vi "main 5th.vi"() -> ()   [LabVIEW 2015]
panel:
  out "data":u16[](array[numeric])
  out "size(s)":i32
  in  "bstrFilename":string
  out "Array":u16[][](array[numeric])
  out "element":u16[][](array[numeric])
  out "From OD fit?":bool
  in  "Current file num":i32
  in  "Fitting Results Save Path":string[](array[string])
  in  "Initial guess values":dbl[](array[numeric])
  out "Latest image data":dbl[][](array[numeric])
  in  "Fitting Type":u16(ring)
  in  "Force Guess?":bool
  out "x-y":u32
  out "best fit parameters":dbl[](array[numeric])
  in  "Reset process index":bool
  out "ROI Height":u32
  out "ROI Width":u32
  out "OD image":u16[][](graph)
  out "Process Index":i32
  out "External Trigger":bool
  out "XY图":cluster{i32[], dbl[]}[](graph)
  in  "OD fit":bool
  in  "OD num":i32
  out "Fit Done":bool
  in  "Exit":bool
  out "XY图 2":cluster{i32[], dbl[]}[](graph)
  in  "Fit":bool
  in  "Open File":bool
  in  "Auto Fit":bool
  in  "Stop":bool
  in  "Aquire":bool
  in  "Fitting Config":bool
  in  "Camera Config":bool
  in  "Initialize":bool
  in  "Live Image Display":refnum<k7>(container)
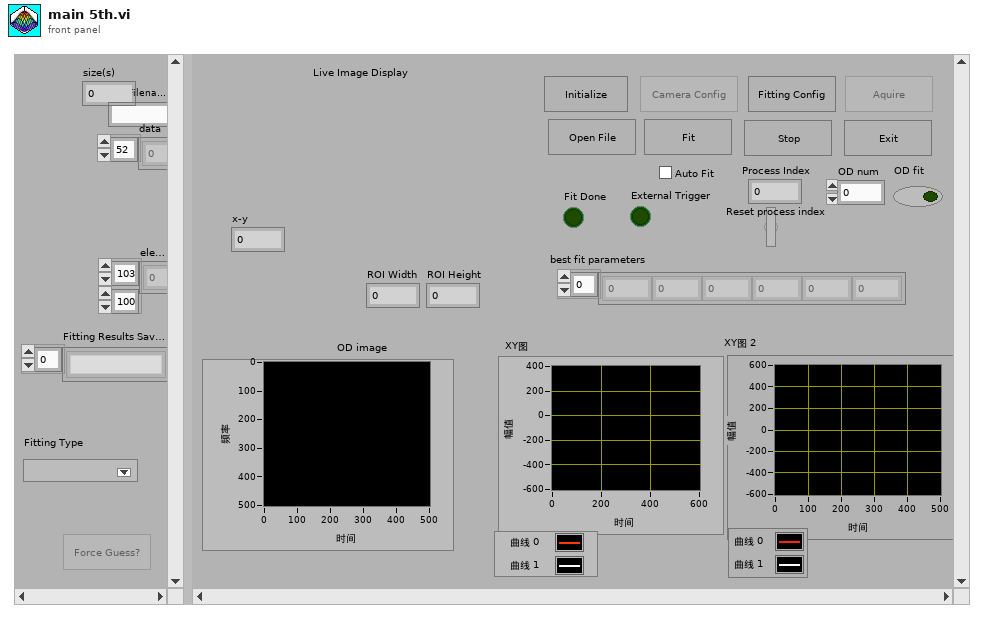
[diagram p1: front panel]
types:
  T1 = enum8{"Enabled", "Disabled", "Disabled and Grayed Out"}
  T2 = typedef "Image Type" = u32
  T3 = typedef "IMAQ Image.ctl" = refnum<image>
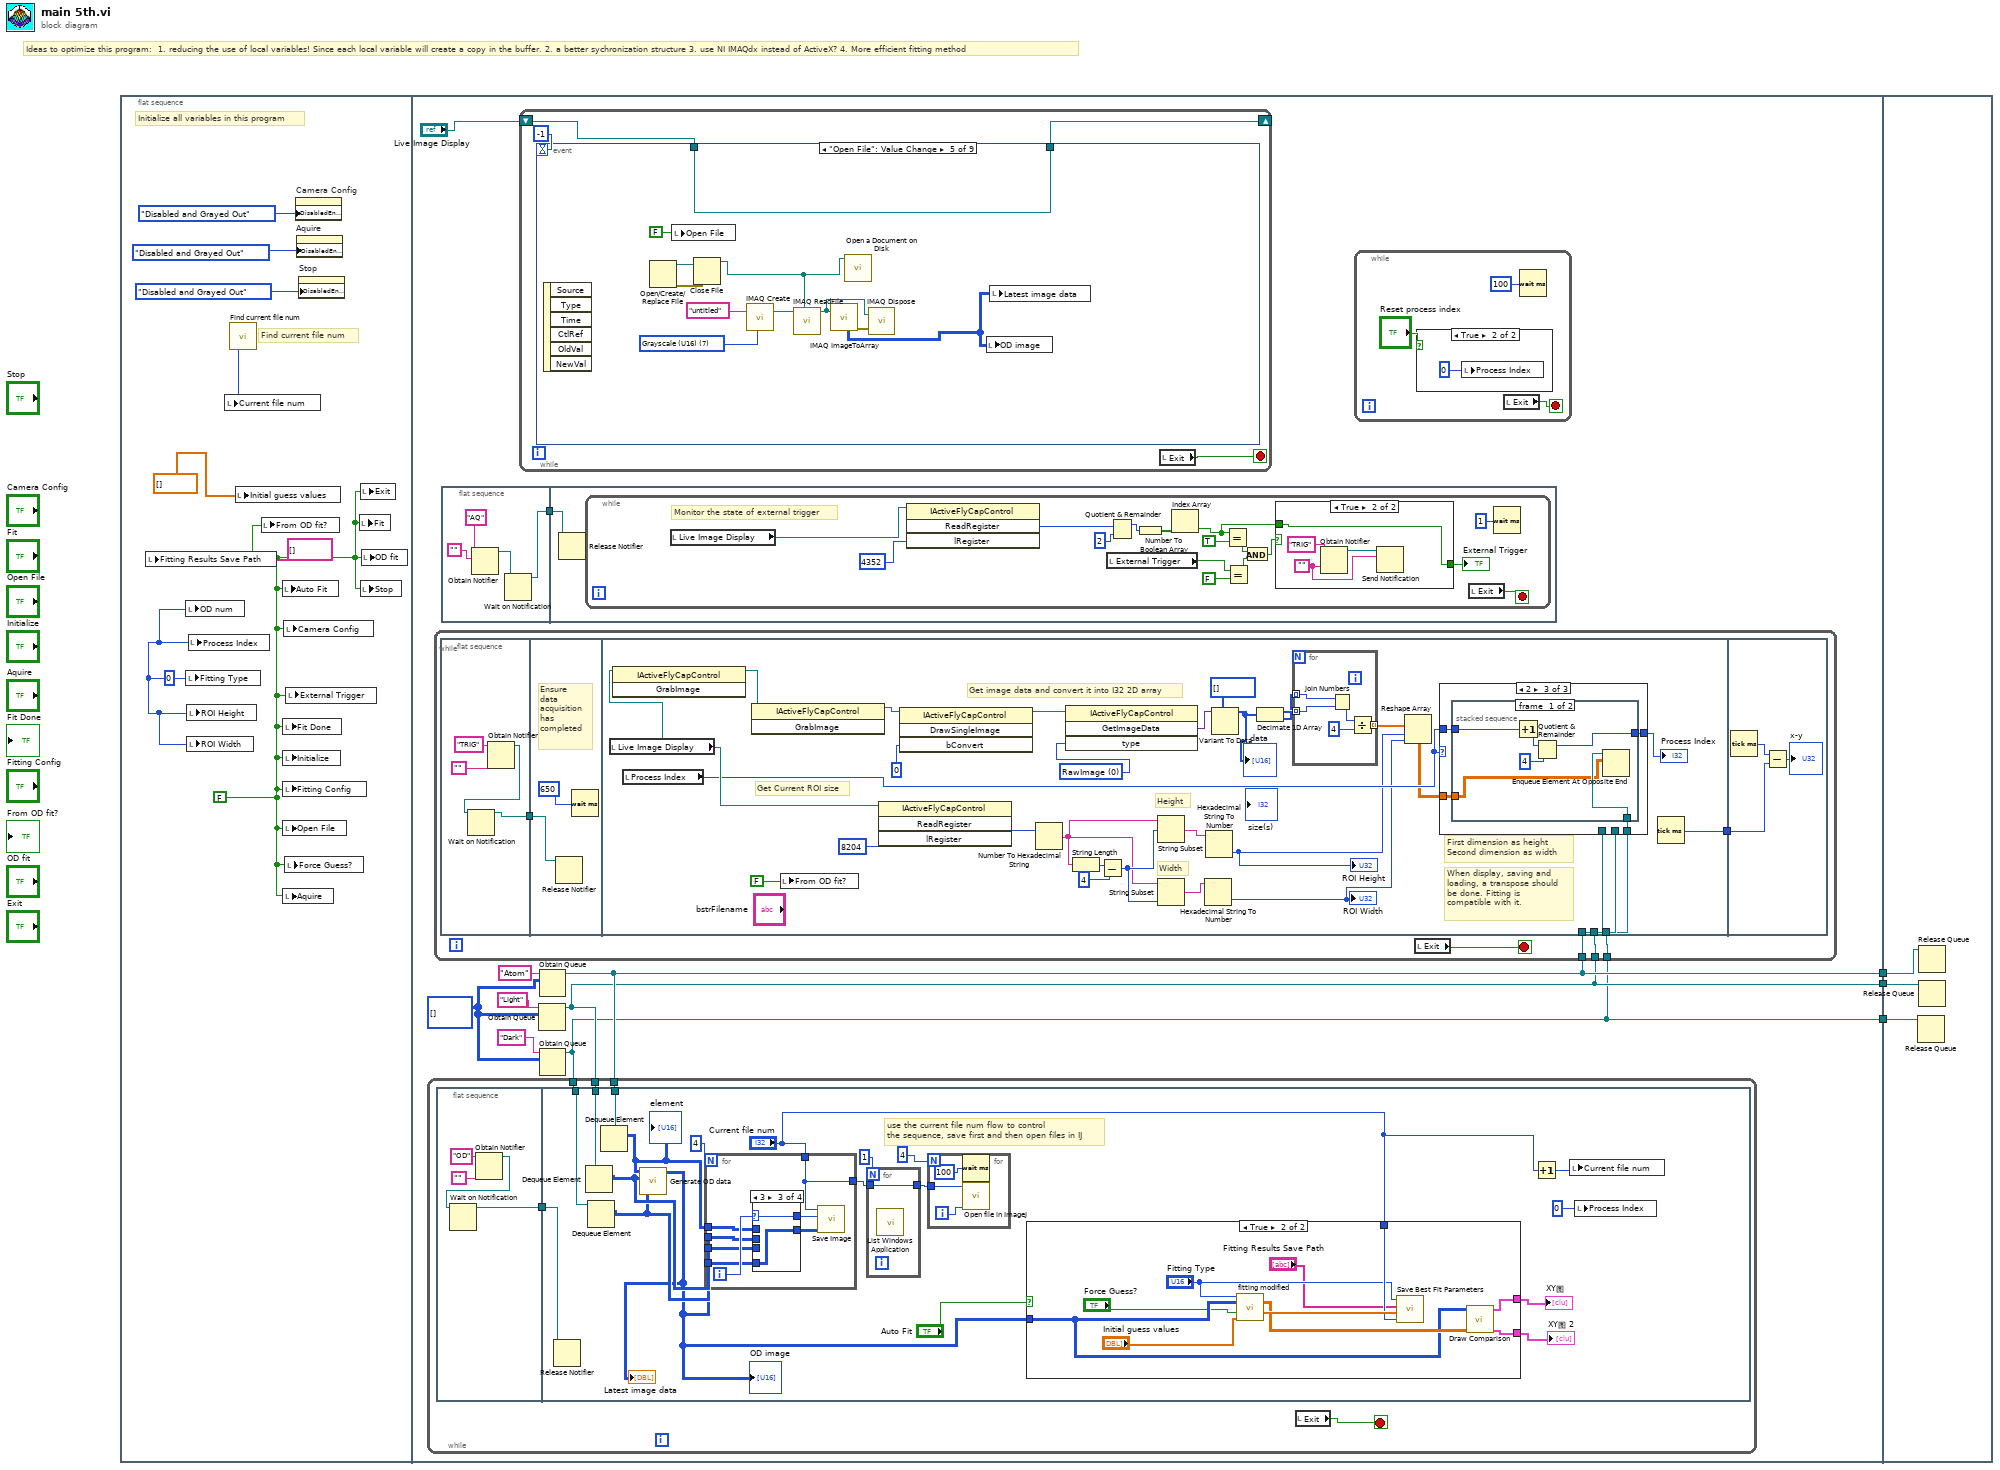
[diagram p0: block diagram]
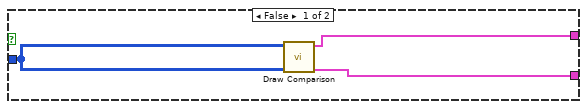
[diagram p3: hidden frame]
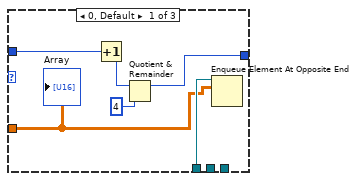
[diagram p8: hidden frame]
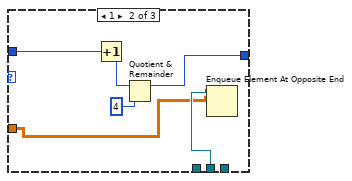
[diagram p9: hidden frame]
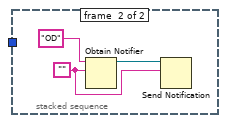
[diagram p10: hidden frame]
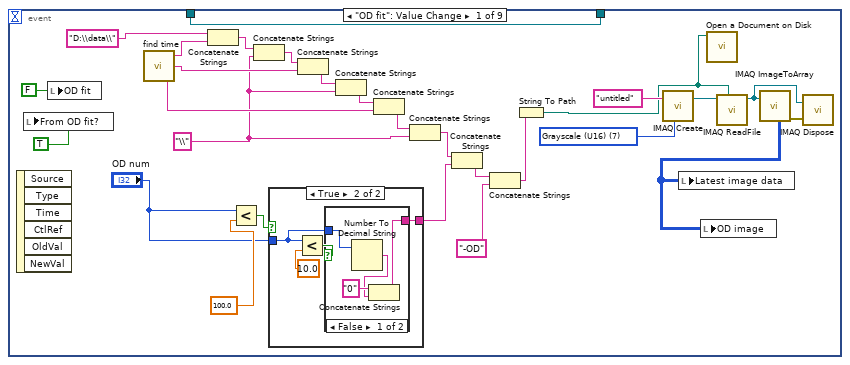
[diagram p11: hidden frame]
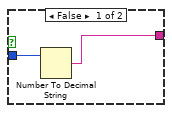
[diagram p12: hidden frame]
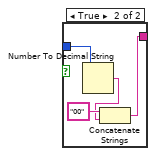
[diagram p13: hidden frame]
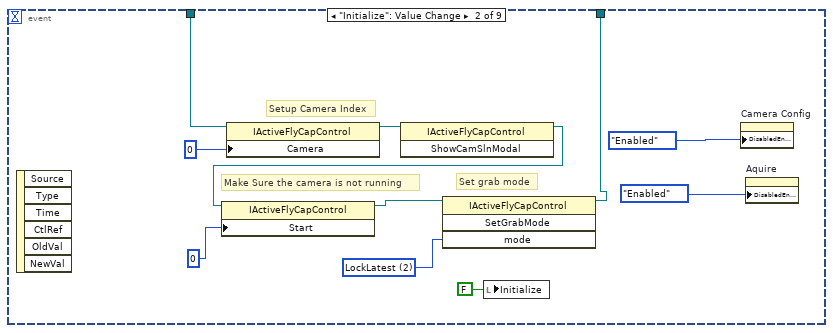
[diagram p14: hidden frame]
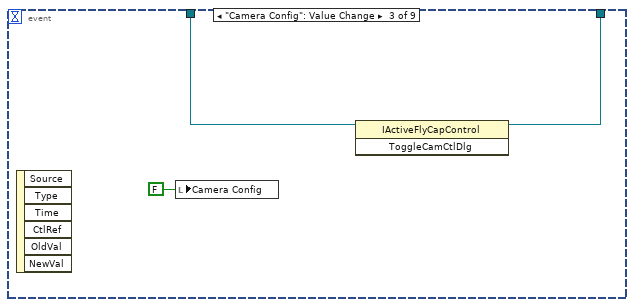
[diagram p15: hidden frame]
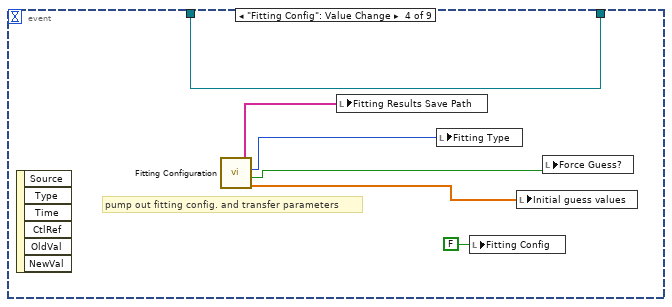
[diagram p16: hidden frame]
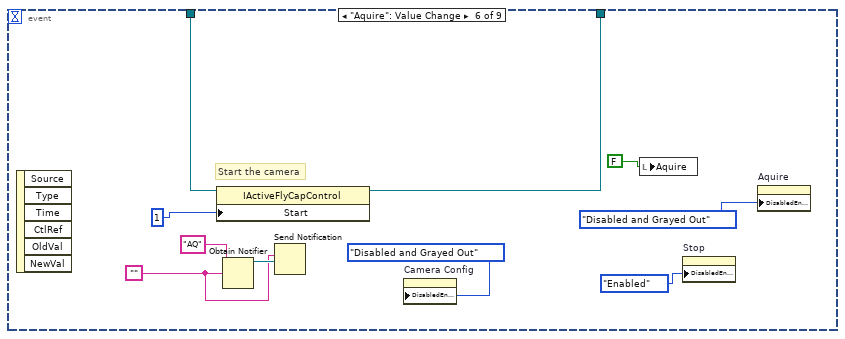
[diagram p17: hidden frame]
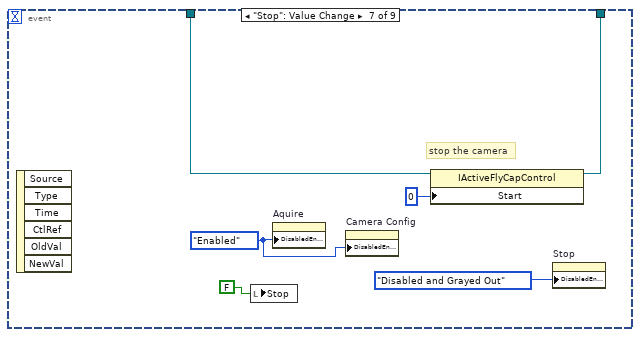
[diagram p18: hidden frame]
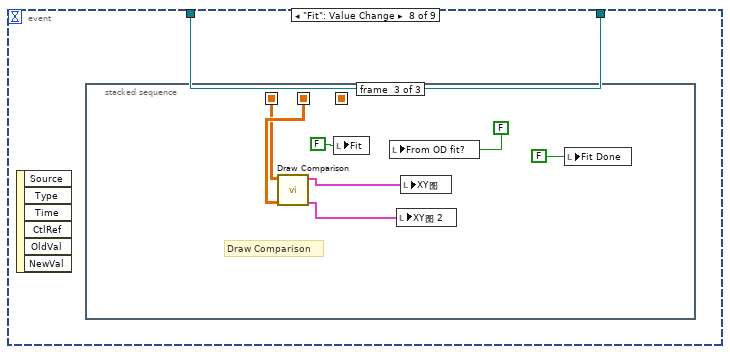
[diagram p19: hidden frame]
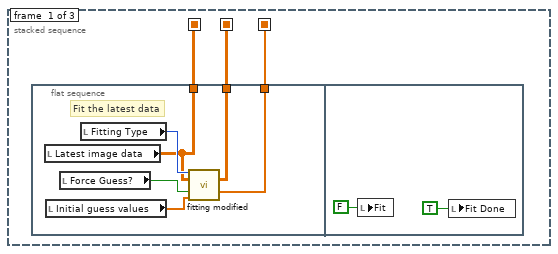
[diagram p20: hidden frame]
diagram:
  # "Ideas to optimize this program:  1. reducing the use of local variables! Since each local variable will create a copy in the buffer. 2. a better sychronization structure 3. use NI IMAQdx instead of ActiveX? 4. More efficient fitting method"
  n1 = flat-sequence {
    tunnel: [w15] -> w3
    tunnel: [w14] -> w2
    tunnel: [w13] -> w1
    tunnel: w3 -> [w309]
    tunnel: w2 -> [w308]
    tunnel: w1 -> [w307]
    frame #0 {
      w7 = 0 ("OD num")
      w5 = FALSE ("Aquire")
      # "Find current file num"
      # "Initialize all variables in this program"
      n2 = local write "Fitting Results Save Path"(string[] [] ("Fitting Results Save Path")) -> ()
      n3 = local write "OD num"(w7) -> ()
      n4 = local write "Fitting Type"(w7) -> ()
      n5 = local write "ROI Height"(w7) -> ()
      n6 = local write "ROI Width"(w7) -> ()
      n7 = local write "Process Index"(w7) -> ()
      n8 = call "Find current file num.vi"() -> ("Current File Num"=w4:u16)  [unwired: 2 in]
      n9 = local write "Current file num"(w4) -> ()
      n10 = local write "Initial guess values"(dbl[] [] ("Best fit parameters")) -> ()
      n11 = local write "From OD fit?"(w5) -> ()
      n12 = local write "Auto Fit"(w5) -> ()
      n13 = local write "Fit Done"(w5) -> ()
      n14 = local write "Initialize"(w5) -> ()
      n15 = local write "Fitting Config"(w5) -> ()
      n16 = local write "Open File"(w5) -> ()
      n17 = local write "Aquire"(w5) -> ()
      n18 = local write "Camera Config"(w5) -> ()
      n19 = local write "Force Guess?"(w5) -> ()
      n20 = local write "External Trigger"(w5) -> ()
      n21 = property on="Camera Config" class="Bool (strict)"("DisabledEnum"=T1."Disabled and Grayed Out" ("禁用")) -> ()  [unwired: 2 in, 2 out]
      n22 = property on="Aquire" class="Bool (strict)"("DisabledEnum"=T1."Disabled and Grayed Out" ("禁用")) -> ()  [unwired: 2 in, 2 out]
      n23 = property on="Stop" class="Bool (strict)"("DisabledEnum"=T1."Disabled and Grayed Out" ("禁用")) -> ()  [unwired: 2 in, 2 out]
      n24 = local write "Fit"(w5) -> ()
      n25 = local write "Exit"(w5) -> ()
      n26 = local write "Stop"(w5) -> ()
      n27 = local write "OD fit"(w5) -> ()
    }
    frame #1 {
      w16 = i32[][] [] ("输出数组")
      n28 = flat-sequence {
        tunnel: [w86] -> w20
        tunnel: w20 -> [w90]
        frame #0 {
          n29 = Obtain Notifier(name (unnamed)="AQ" ("名称（未命名）"), notification data type="") -> (notifier out=w88:refnum<notifier>)  [unwired: 2 in, 2 out]
          n30 = Wait on Notification(notifier=w88) -> (notifier out=w86:refnum<notifier>)  [unwired: 3 in, 3 out]
        }
        frame #1 {
          n31 = Release Notifier(notifier=w90) -> ()  [unwired: 2 in, 3 out]
          n32 = while {
            stop <- w106 stop-if-true
            # "Monitor the state of external trigger"
            n33 = local read "Live Image Display"() -> (w105:refnum<k7>)
            n34 = invoke class="IActiveFlyCapControl" method="ReadRegister"(reference=w105, "lRegister"=u32 4352) -> ("ReadRegister"=w103:u32)  [unwired: 2 in, 3 out]
            n35 = local read "External Trigger"() -> (w98:bool)
            n36 = Quotient & Remainder(x=w103, y=u32 2) -> (x-y*floor(x/y)=w101:u32)  [unwired: 1 out]
            n37 = Number To Boolean Array(number=w101) -> (Boolean array=w100:bool[])
            n38 = Index Array(array=w100) -> (element=w93:bool)  [unwired: 1 in]
            n39 = Equal?(x=w93, y=TRUE) -> (x = y?=w95:bool)
            n40 = Equal?(x=w98, y=FALSE) -> (x = y?=w96:bool)
            n41 = And(x=w95, y=w96) -> (x .and. y?=w94:bool)
            n42 = case shown="True" w94 {
              tunnel: w93 -> [w107 w108]
              tunnel: [w107 w108] -> w91
              frame False {
              }
              frame True {
                w109 = ""
                n43 = Obtain Notifier(name (unnamed)="TRIG" ("名称（未命名）"), notification data type=w109) -> (notifier out=w110:refnum<notifier>)  [unwired: 2 in, 2 out]
                n44 = Send Notification(notification=w109, notifier=w110) -> ()  [unwired: 1 in, 2 out]
              }
            }
            "External Trigger" <- w91
            n45 = local read "Exit"() -> (w106:bool)
            n46 = Wait (ms)(milliseconds to wait=u32 1 ("等待时间（毫秒）")) -> ()  [unwired: 1 out]
          }
        }
      }
      n47 = while {
        shift-right: [w187] -> _
        shift-left: "Live Image Display" -> [w188]
        stop <- w190 stop-if-true
        n48 = event shown="[4] \"Open File\": Value Change" {
          selector: _ -> [_ _ _ _ _ _ _ _ _]
          dyn-events: _ -> [_ _ _ _ _ _ _ _ _]
          timeout: -1 -> [_ _ _ _ _ _ _ _ _]
          tunnel: w188 -> [w216 w237 w245 w247 w262 w265 w276 w280 w306]
          tunnel: [w216 w233 w244 w247 w262 w264 w275 w280 w306] -> w187
          event "OD fit": Value Change {
            w197 = T2 7 items=["Grayscale (U8)", "Grayscale (I16)", "Grayscale (SGL)", "Complex (CSG)", "RGB (U32)", "HSL (U32)", "RGB (U64)", "Grayscale (U16)"] ("Image Type")
            w206 = "\\" ("字符串")
            n49 = event-data() -> ()  [unwired: 1 in, 6 out]
            n50 = local write "From OD fit?"(TRUE ("From OD fit?")) -> ()
            n51 = local write "OD fit"(FALSE ("OD fit")) -> ()
            n52 = call "find time.vi"() -> ("day"=w208:string, "month"=w211:string, "year"=w214:string)  [unwired: 3 in]
            n53 = Concatenate Strings("D:\\data\\", w214) -> (w213:string)
            n54 = Less?(x="OD num", y=100.0) -> (x < y?=w200:bool)
            n55 = Concatenate Strings(w213, w206) -> (w212:string)
            n56 = case shown="True" w200 {
              tunnel: "OD num" -> [w220 w222]
              tunnel: [w219 w221] -> w199
              frame False {
                n57 = Number To Decimal String(number=w220) -> (decimal integer string=w219:string)  [unwired: 1 in]
              }
              frame True {
                n58 = Less?(x=w222, y=10.0) -> (x < y?=w223:bool)
                n59 = case shown="False" w223 {
                  tunnel: w222 -> [w227 w232]
                  tunnel: [w225 w229] -> w221
                  frame False {
                    n60 = Number To Decimal String(number=w227) -> (decimal integer string=w226:string)  [unwired: 1 in]
                    n61 = Concatenate Strings("0" ("字符串"), w226) -> (w225:string)
                  }
                  frame True {
                    n62 = Number To Decimal String(number=w232) -> (decimal integer string=w230:string)  [unwired: 1 in]
                    n63 = Concatenate Strings("00" ("字符串"), w230) -> (w229:string)
                  }
                }
              }
            }
            n64 = Concatenate Strings(w212, w211) -> (w210:string)
            n65 = Concatenate Strings(w210, w206) -> (w209:string)
            n66 = Concatenate Strings(w209, w208) -> (w207:string)
            n67 = Concatenate Strings(w207, w206) -> (w205:string)
            n68 = Concatenate Strings(w205, w199) -> (w204:string)
            n69 = Concatenate Strings(w204, "-OD" ("字符串")) -> (w202:string)
            n70 = String To Path(string=w202) -> (path=w193:path)
            n71 = call "IMAQ Create"("Image Name"="untitled", "Image Type"=w197) -> ("New Image"=w192:T3)  [unwired: 3 in, 1 out]
            n72 = call <vilib>:"Open a Document on Disk.vi"("document path"=w193) -> ()  [unwired: 6 in, 1 out]
            n73 = call "IMAQ ReadFile"("File Path"=w193, "Image"=w192) -> ("Image Out"=w191:T3)  [unwired: 5 in, 4 out]
            n74 = call "IMAQ ImageToArray"("Image"=w191) -> ("Image Pixels (U16)"=w195:u16[][], "error out"=w196:errorcluster)  [unwired: 3 in, 3 out]
            n75 = local write "Latest image data"(w195) -> ()
            n76 = local write "OD image"(w195) -> ()
            n77 = call "IMAQ Dispose"("Image"=w191, "error in (no error)"=w196) -> ()  [unwired: 4 in, 1 out]
          }
          event "Initialize": Value Change {
            w241 = 2 items=["FreeRunning", "LockNext", "LockLatest"] ("mode")
            # "Setup Camera Index"
            # "Set grab mode"
            # "Make Sure the camera is not running"
            n78 = event-data() -> ()  [unwired: 1 in, 6 out]
            n79 = property class="IActiveFlyCapControl"(reference=w237, "Camera"=0 ("Start")) -> (reference out=w240:refnum<k7>)  [unwired: 1 in, 1 out]
            n80 = invoke class="IActiveFlyCapControl" method="ShowCamSlnModal"(reference=w240) -> (reference out=w236:refnum<k7>)  [unwired: 2 in, 2 out]
            n81 = property class="IActiveFlyCapControl"(reference=w236, "Start"=0 ("Camera")) -> (reference out=w235:refnum<k7>)  [unwired: 1 in, 1 out]
            n82 = invoke class="IActiveFlyCapControl" method="SetGrabMode"(reference=w235, "mode"=w241) -> (reference out=w233:refnum<k7>)  [unwired: 2 in, 3 out]
            n83 = local write "Initialize"(FALSE ("Initialize")) -> ()
            n84 = property on="Camera Config" class="Bool (strict)"("DisabledEnum"=T1."Enabled" ("禁用")) -> ()  [unwired: 2 in, 2 out]
            n85 = property on="Aquire" class="Bool (strict)"("DisabledEnum"=T1."Enabled" ("禁用")) -> ()  [unwired: 2 in, 2 out]
          }
          event "Camera Config": Value Change {
            n86 = event-data() -> ()  [unwired: 1 in, 6 out]
            n87 = local write "Camera Config"(FALSE ("Camera Config")) -> ()
            n88 = invoke class="IActiveFlyCapControl" method="ToggleCamCtlDlg"(reference=w245) -> (reference out=w244:refnum<k7>)  [unwired: 2 in, 2 out]
          }
          event "Fitting Config": Value Change {
            # "pump out fitting config. and transfer parameters"
            n89 = event-data() -> ()  [unwired: 1 in, 6 out]
            n90 = call "Fitting Configuration.vi"() -> ("intial guess"=w248:dbl[], "Force Guess？"=w249:bool, "Fitting Type"=w251:u16, "Fitting Results Save Path"=w250:string[])  [unwired: 5 in]
            n91 = local write "Fitting Results Save Path"(w250) -> ()
            n92 = local write "Fitting Type"(w251) -> ()
            n93 = local write "Fitting Config"(FALSE ("Fitting Config")) -> ()
            n94 = local write "Initial guess values"(w248) -> ()
            n95 = local write "Force Guess?"(w249) -> ()
          }
          event "Open File": Value Change {
            w261 = T2 7 items=["Grayscale (U8)", "Grayscale (I16)", "Grayscale (SGL)", "Complex (CSG)", "RGB (U32)", "HSL (U32)", "RGB (U64)", "Grayscale (U16)"] ("Image Type")
            n96 = event-data() -> ()  [unwired: 1 in, 6 out]
            n97 = Open/Create/Replace File() -> (refnum out=w254:refnum<file>, error out=w255:errorcluster)  [unwired: 6 in, 1 out]
            n98 = local write "Open File"(FALSE ("Open File")) -> ()
            n99 = Close File(refnum=w254, error in=w255) -> (path=w253:path)  [unwired: 1 out]
            n100 = call "IMAQ Create"("Image Name"="untitled", "Image Type"=w261) -> ("New Image"=w260:T3)  [unwired: 3 in, 1 out]
            n101 = call "IMAQ ReadFile"("File Path"=w253, "Image"=w260) -> ("Image Out"=w259:T3)  [unwired: 5 in, 4 out]
            n102 = call "IMAQ ImageToArray"("Image"=w259) -> ("Image Pixels (U16)"=w256:u16[][], "error out"=w258:errorcluster)  [unwired: 3 in, 3 out]
            n103 = call <vilib>:"Open a Document on Disk.vi"("document path"=w253) -> ()  [unwired: 6 in, 1 out]
            n104 = call "IMAQ Dispose"("Image"=w259, "error in (no error)"=w258) -> ()  [unwired: 4 in, 1 out]
            n105 = local write "OD image"(w256) -> ()
            n106 = local write "Latest image data"(w256) -> ()
          }
          event "Aquire": Value Change {
            w267 = ""
            # "Start the camera"
            n107 = event-data() -> ()  [unwired: 1 in, 6 out]
            n108 = property class="IActiveFlyCapControl"(reference=w265, "Start"=1) -> (reference out=w264:refnum<k7>)  [unwired: 1 in, 1 out]
            n109 = Obtain Notifier(name (unnamed)="AQ" ("名称（未命名）"), notification data type=w267) -> (notifier out=w268:refnum<notifier>)  [unwired: 2 in, 2 out]
            n110 = Send Notification(notification=w267, notifier=w268) -> ()  [unwired: 1 in, 2 out]
            n111 = property on="Camera Config" class="Bool (strict)"("DisabledEnum"=T1."Disabled and Grayed Out" ("禁用")) -> ()  [unwired: 2 in, 2 out]
            n112 = local write "Aquire"(FALSE ("Initialize")) -> ()
            n113 = property on="Stop" class="Bool (strict)"("DisabledEnum"=T1."Enabled" ("禁用")) -> ()  [unwired: 2 in, 2 out]
            n114 = property on="Aquire" class="Bool (strict)"("DisabledEnum"=T1."Disabled and Grayed Out" ("禁用")) -> ()  [unwired: 2 in, 2 out]
          }
          event "Stop": Value Change {
            w274 = T1."Enabled" ("禁用")
            # "stop the camera"
            n115 = event-data() -> ()  [unwired: 1 in, 6 out]
            n116 = local write "Stop"(FALSE ("Initialize")) -> ()
            n117 = property on="Aquire" class="Bool (strict)"("DisabledEnum"=w274) -> ()  [unwired: 2 in, 2 out]
            n118 = property on="Camera Config" class="Bool (strict)"("DisabledEnum"=w274) -> ()  [unwired: 2 in, 2 out]
            n119 = property class="IActiveFlyCapControl"(reference=w276, "Start"=0) -> (reference out=w275:refnum<k7>)  [unwired: 1 in, 1 out]
            n120 = property on="Stop" class="Bool (strict)"("DisabledEnum"=T1."Disabled and Grayed Out" ("禁用")) -> ()  [unwired: 2 in, 2 out]
          }
          event "Fit": Value Change {
            n121 = event-data() -> ()  [unwired: 1 in, 6 out]
            n122 = stacked-sequence {
              seq-local: [w282 _ _] -> [_ _ w302]
              seq-local: [w283 _ _] -> [_ _ w300]
              seq-local: [w281 _ _] -> [_ w292 _]
              frame #0 {
                n123 = flat-sequence {
                  tunnel: [w286] -> w283
                  tunnel: [w285] -> w282
                  tunnel: [w284] -> w281
                  frame #0 {
                    # "Fit the latest data"
                    n124 = local read "Latest image data"() -> (w286:dbl[][])
                    n125 = local read "Initial guess values"() -> (w288:dbl[])
                    n126 = local read "Force Guess?"() -> (w289:bool)
                    n127 = local read "Fitting Type"() -> (w287:u16)
                    n128 = call "fitting modified.vi"("fitting type"=w287, "2D data"=w286, "force guess?"=w289, "intial guess value"=w288) -> ("best fit"=w285:dbl[][], "best fit parameters"=w284:dbl[])  [unwired: 8 in, 2 out]
                  }
                  frame #1 {
                    n129 = local write "Fit"(FALSE ("Fit")) -> ()
                    n130 = local write "Fit Done"(TRUE ("Fit Done")) -> ()
                  }
                }
              }
              frame #1 {
                # "Save best fit parameters"
                n131 = local read "Fitting Results Save Path"() -> (w295:string[])
                n132 = local read "Fitting Type"() -> (w296:u16)
                n133 = local read "From OD fit?"() -> (w294:bool)
                n134 = case shown="True" w294 {
                  tunnel: [w297 w298] -> w293
                  frame False {
                    n135 = local read "Current file num"() -> (w297:i32)
                  }
                  frame True {
                    n136 = local read "OD num"() -> (w298:i32)
                  }
                }
                n137 = call "Save Best Fit Parameters.vi"("Current File Num"=w293, "Best Fit Parameters"=w292, "Fitting Results Save Path"=w295, "Fitting Type"=w296) -> ()  [unwired: 8 in]
                "best fit parameters" <- w292
              }
              frame #2 {
                # "Draw Comparison"
                n138 = call "Draw Comparison.vi"("Best Fit"=w302, "Raw Data"=w300) -> ("Vertical Comparison"=w304:cluster{i32[], dbl[]}[], "Horizontal Comparison"=w305:cluster{i32[], dbl[]}[])  [unwired: 7 in]
                n139 = local write "Fit"(FALSE ("Initialize")) -> ()
                n140 = local write "From OD fit?"(FALSE ("From OD fit?")) -> ()
                n141 = local write "XY图 2"(w304) -> ()
                n142 = local write "XY图"(w305) -> ()
                n143 = local write "Fit Done"(FALSE ("Fit Done")) -> ()
              }
            }
          }
          event Timeout {
            n144 = event-data() -> ()  [unwired: 1 in, 3 out]
          }
        }
        n145 = local read "Exit"() -> (w190:bool)
      }
      n146 = Obtain Queue(name (unnamed)="Light" ("名称（未命名）"), element data type=w16) -> (queue out=w14:refnum<queue>)  [unwired: 3 in, 2 out]
      n147 = Obtain Queue(name (unnamed)="Atom" ("名称（未命名）"), element data type=w16) -> (queue out=w15:refnum<queue>)  [unwired: 3 in, 2 out]
      n148 = Obtain Queue(name (unnamed)="Dark" ("名称（未命名）"), element data type=w16) -> (queue out=w13:refnum<queue>)  [unwired: 3 in, 2 out]
      n149 = while {
        tunnel: w15 -> [w27]
        tunnel: w14 -> [w26]
        tunnel: w13 -> [w25]
        stop <- w29 stop-if-true
        n150 = flat-sequence {
          tunnel: [w30] -> w28
          tunnel: w28 -> [w52]
          tunnel: w27 -> [w50]
          tunnel: w26 -> [w48]
          tunnel: w25 -> [w46]
          frame #0 {
            n151 = Obtain Notifier(name (unnamed)="OD" ("名称（未命名）"), notification data type="") -> (notifier out=w31:refnum<notifier>)  [unwired: 2 in, 2 out]
            n152 = Wait on Notification(notifier=w31) -> (notifier out=w30:refnum<notifier>)  [unwired: 3 in, 3 out]
          }
          frame #1 {
            # "use the current file num flow to control \nthe sequence, save first and then open files in IJ"
            n153 = Release Notifier(notifier=w52) -> ()  [unwired: 2 in, 3 out]
            n154 = Dequeue Element(queue=w48) -> (element=w47:i32[][])  [unwired: 2 in, 3 out]
            n155 = Dequeue Element(queue=w46) -> (element=w45:i32[][])  [unwired: 2 in, 3 out]
            n156 = Dequeue Element(queue=w50) -> (element=w49:i32[][])  [unwired: 2 in, 3 out]
            "element" <- w49
            n157 = call "Generate OD data.vi"("dark"=w45, "light"=w47, "atom"=w49) -> ("OD image"=w41:u16[][])  [unwired: 3 in]
            "OD image" <- w41
            "Latest image data" <- w41
            n158 = for {
              N: 4 -> [_]
              tunnel: w49 -> [w76]
              tunnel: w47 -> [w75]
              tunnel: w45 -> [w74]
              tunnel: w41 -> [w73]
              tunnel: "Current file num" -> [w70]
              tunnel: [w70] -> w34
              i -> [w77]
              n159 = case shown="3" w77 {
                selector: w77 -> [w79 w81 w83 w85]
                tunnel: w76 -> [w78 _ _ _]
                tunnel: w75 -> [_ _ _ w84]
                tunnel: w74 -> [_ w80 _ _]
                tunnel: w73 -> [_ _ w82 _]
                tunnel: [w79 w81 w83 w85] -> w72
                tunnel: [w78 w80 w82 w84] -> w71
                frame 0, Default {
                }
                frame 2 {
                }
                frame 3 {
                }
                frame 1 {
                }
              }
              n160 = call "Save Image.vi"("Data"=w71, "Process Index"=w72, "Current File Num"=w70) -> ()  [unwired: 9 in]
            }
            n161 = for {
              N: 1 -> [_]
              tunnel: w34 -> [w53]
              tunnel: [w53] -> w36
              n162 = call "List Windows Application.vi"() -> ()  [unwired: 1 in]
            }
            n163 = for {
              N: 4 -> [_]
              tunnel: w36 -> [w56]
              i -> [w55]
              n164 = Wait (ms)(milliseconds to wait=u32 100) -> ()  [unwired: 1 out]
              n165 = call "Open file in ImageJ.vi"("Process Index"=w55, "Current File Num"=w56) -> ()  [unwired: 10 in]
            }
            n166 = case shown="True" "Auto Fit" {
              tunnel: w41 -> [w59 w66]
              tunnel: "Current file num" -> [_ w68]
              tunnel: [w58 w65] -> w42
              tunnel: [w57 w64] -> w43
              frame False {
                n167 = call "Draw Comparison.vi"("Best Fit"=w59, "Raw Data"=w59) -> ("Vertical Comparison"=w57:cluster{i32[], dbl[]}[], "Horizontal Comparison"=w58:cluster{i32[], dbl[]}[])  [unwired: 7 in]
              }
              frame True {
                n168 = call "fitting modified.vi"("fitting type"="Fitting Type", "2D data"=w66, "force guess?"="Force Guess?", "intial guess value"="Initial guess values") -> ("best fit"=w67:dbl[][], "best fit parameters"=w69:dbl[])  [unwired: 8 in, 2 out]
                n169 = call "Save Best Fit Parameters.vi"("Current File Num"=w68, "Best Fit Parameters"=w69, "Fitting Results Save Path"="Fitting Results Save Path", "Fitting Type"="Fitting Type") -> ()  [unwired: 8 in]
                n170 = call "Draw Comparison.vi"("Best Fit"=w67, "Raw Data"=w66) -> ("Vertical Comparison"=w64:cluster{i32[], dbl[]}[], "Horizontal Comparison"=w65:cluster{i32[], dbl[]}[])  [unwired: 7 in]
              }
            }
            "XY图" <- w42
            "XY图 2" <- w43
            n171 = Increment(x="Current file num") -> (x+1=w40:i32)
            n172 = local write "Current file num"(w40) -> ()
            n173 = local write "Process Index"(0 ("Process Index")) -> ()
          }
        }
        n174 = local read "Exit"() -> (w29:bool)
      }
      n175 = while {
        tunnel: w15 -> [w115]
        tunnel: w14 -> [w114]
        tunnel: w13 -> [w113]
        stop <- w117 stop-if-true
        n176 = flat-sequence {
          tunnel: [w118] -> w116
          tunnel: w116 -> [w123]
          tunnel: w115 -> [w137]
          tunnel: w114 -> [w136]
          tunnel: w113 -> [w135]
          tunnel: [w124] -> w112
          tunnel: w112 -> [w185]
          frame #0 {
            n177 = Obtain Notifier(name (unnamed)="TRIG" ("名称（未命名）"), notification data type="") -> (notifier out=w119:refnum<notifier>)  [unwired: 2 in, 2 out]
            n178 = Wait on Notification(notifier=w119) -> (notifier out=w118:refnum<notifier>)  [unwired: 3 in, 3 out]
          }
          frame #1 {
            # "Ensure\ndata\nacquisition\nhas \ncompleted"
            n179 = Release Notifier(notifier=w123) -> ()  [unwired: 2 in, 3 out]
            n180 = Wait (ms)(milliseconds to wait=u32 650 ("等待时间（毫秒）")) -> ()  [unwired: 1 out]
          }
          frame #2 {
            w153 = 0 items=["RawImage", "ColorProcessedImage"] ("type")
            # "Get image data and convert it into I32 2D array"
            # "When display, saving and \nloading, a transpose should\nbe done. Fitting is \ncompatible with it."
            # "First dimension as height\nSecond dimension as width"
            # "Width"
            # "Height"
            # "Get Current ROI size"
            n181 = local read "Live Image Display"() -> (w142:refnum<k7>)
            n182 = invoke class="IActiveFlyCapControl" method="GrabImage"(reference=w142) -> (reference out=w126:refnum<k7>)  [unwired: 2 in, 2 out]
            n183 = local read "Process Index"() -> (w139:i32)
            n184 = invoke class="IActiveFlyCapControl" method="GrabImage"(reference=w126) -> (reference out=w125:refnum<k7>)  [unwired: 2 in, 2 out]
            n185 = local write "From OD fit?"(FALSE ("From OD fit?")) -> ()
            n186 = invoke class="IActiveFlyCapControl" method="ReadRegister"(reference=w142, "lRegister"=u32 8204) -> ("ReadRegister"=w151:u32)  [unwired: 2 in, 3 out]
            n187 = invoke class="IActiveFlyCapControl" method="DrawSingleImage"(reference=w125, "bConvert"=0) -> (reference out=w141:refnum<k7>)  [unwired: 2 in, 3 out]
            n188 = Number To Hexadecimal String(2:w151) -> (0:w147:string)  [unwired: 1 in]
            n189 = invoke class="IActiveFlyCapControl" method="GetImageData"(reference=w141, "type"=w153) -> ("GetImageData"=w133:variant)  [unwired: 2 in, 3 out]
            n190 = String Length(string=w147) -> (length=w150:i32)
            n191 = Subtract(x=w150, y=4) -> (x-y=w148:i32)
            n192 = String Subset(string=w147, length (rest)=w148) -> (substring=w144:string)  [unwired: 1 in]
            n193 = String Subset(string=w147, offset (0)=w148) -> (substring=w145:string)  [unwired: 1 in]
            n194 = Hexadecimal String To Number(string=w144) -> (number=w131:u32)  [unwired: 2 in, 1 out]
            "ROI Width" <- w131
            n195 = Hexadecimal String To Number(string=w145) -> (number=w132:u32)  [unwired: 2 in, 1 out]
            "ROI Height" <- w132
            n196 = Variant To Data(type=u8[] [], Variant=w133) -> (data=w130:u8[])  [unwired: 1 in, 1 out]
            "data" <- w130
            n197 = Decimate 1D Array(w130) -> (w129:u8[], w128:u8[])
            n198 = for {
              tunnel: w129 -> [w157] mode=indexing
              tunnel: w128 -> [w158] mode=indexing
              tunnel: [w154] -> w127 mode=indexing
              n199 = Join Numbers(hi=w158, lo=w157) -> ((hi.lo)=w156:u16)
              n200 = Divide(x=w156, y=u16 4) -> (x/y=w154:dbl)
            }
            n201 = Reshape Array(w127, w132, w131) -> (w138:dbl[][])
            n202 = case shown="2" w139 {
              tunnel: w139 -> [w162 w168 w174]
              tunnel: w138 -> [w159 w165 w173]
              tunnel: w137 -> [w160 _ _]
              tunnel: w136 -> [_ w166 _]
              tunnel: w135 -> [_ _ w172]
              tunnel: [w161 w167 w171] -> w134
              frame 0, Default {
                n203 = Increment(x=w162) -> (x+1=w163:i32)
                n204 = Quotient & Remainder(x=w163, y=4) -> (x-y*floor(x/y)=w161:i32)  [unwired: 1 out]
                n205 = Enqueue Element At Opposite End(queue=w160, element=w159) -> ()  [unwired: 2 in, 3 out]
                "Array" <- w159
              }
              frame 1 {
                n206 = Increment(x=w168) -> (x+1=w169:i32)
                n207 = Quotient & Remainder(x=w169, y=4) -> (x-y*floor(x/y)=w167:i32)  [unwired: 1 out]
                n208 = Enqueue Element At Opposite End(queue=w166, element=w165) -> ()  [unwired: 2 in, 3 out]
              }
              frame 2 {
                n209 = stacked-sequence {
                  tunnel: w174 -> [w178 _]
                  tunnel: w173 -> [w175 _]
                  tunnel: w172 -> [w176 _]
                  tunnel: [w177 _] -> w171
                  frame #0 {
                    n210 = Increment(x=w178) -> (x+1=w179:i32)
                    n211 = Quotient & Remainder(x=w179, y=4) -> (x-y*floor(x/y)=w177:i32)  [unwired: 1 out]
                    n212 = Enqueue Element At Opposite End(queue=w176, element=w175) -> ()  [unwired: 2 in, 3 out]
                  }
                  frame #1 {
                    w181 = ""
                    n213 = Obtain Notifier(name (unnamed)="OD" ("名称（未命名）"), notification data type=w181) -> (notifier out=w183:refnum<notifier>)  [unwired: 2 in, 2 out]
                    n214 = Send Notification(notification=w181, notifier=w183) -> ()  [unwired: 1 in, 2 out]
                  }
                }
              }
            }
            "Process Index" <- w134
            n215 = Tick Count (ms)() -> (millisecond timer value=w124:u32)
          }
          frame #3 {
            n216 = Tick Count (ms)() -> (millisecond timer value=w186:u32)
            n217 = Subtract(x=w186, y=w185) -> (x-y=→"x-y":u32)
          }
        }
        n218 = local read "Exit"() -> (w117:bool)
      }
      n219 = while {
        stop <- w23 stop-if-true
        n220 = case shown="True" "Reset process index" {
          frame False {
          }
          frame True {
            n221 = local write "Process Index"(0 ("Process Index")) -> ()
          }
        }
        n222 = local read "Exit"() -> (w23:bool)
        n223 = Wait (ms)(milliseconds to wait=u32 100 ("等待时间（毫秒）")) -> ()  [unwired: 1 out]
      }
    }
    frame #2 {
      n224 = Release Queue(queue=w307) -> ()  [unwired: 2 in, 3 out]
      n225 = Release Queue(queue=w309) -> ()  [unwired: 2 in, 3 out]
      n226 = Release Queue(queue=w308) -> ()  [unwired: 2 in, 3 out]
    }
  }
